vi "超标留样启动流程.vi"   [LabVIEW 2016, in "德润DR803L超标留样.lvlib"]
types:
  T1 = cluster{"采样器状态":enum16{"停止", "运行"}, "当前留样瓶编号":u16, "报警状态":enum16{"无报警", "缺水报警"}, "超标信号":enum16{"无信号", "超标信号"}, "采样器进程":enum16{"停止", "待机", "定位校正", "移除瓶盖", "采样瓶排空", "管路润洗", "管存", "进样", "瓶盖密封", "管路排空", "调整采样位置", "采样结束", "采样瓶润洗", "瓶润洗排空"}, "版本号":string, "同步信号":enum16{"无信号", "同步信号"}, "外控信号":enum16{"无信号", "外控信号"}, "门状态":enum16{"门开", "门关"}, "当前瓶号":u16, "工作状态":enum16{"停止", "采样中"}, "留样模式":enum16{"无", "定时留样", "时间等比例", "超标留样", "同步留样", "外控留样"}, "立即留样":enum16{"无", "远程留样"}, "采样方式":enum16{"单采", "双重"}, "仪器时间":timestamp, "单次采样量":u16, "时间等比采样采样间隔":u16, "排空命令":u16, "远程复位":u16, "门禁密码":u16}
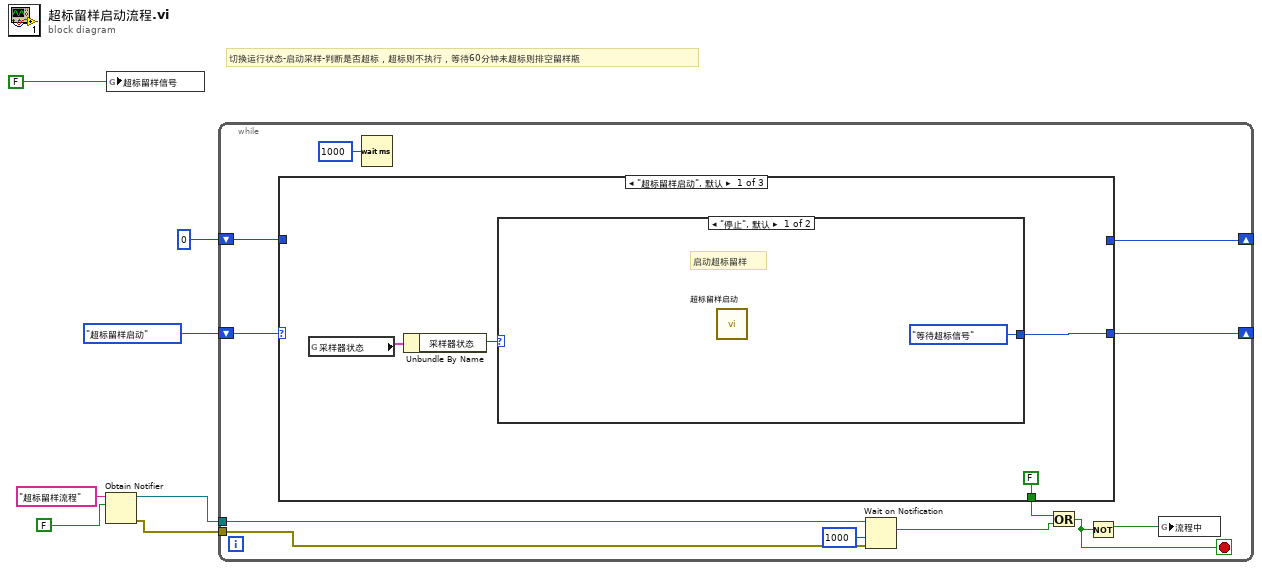
[diagram p0: block diagram]
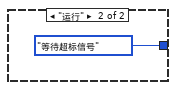
[diagram p2: hidden frame]
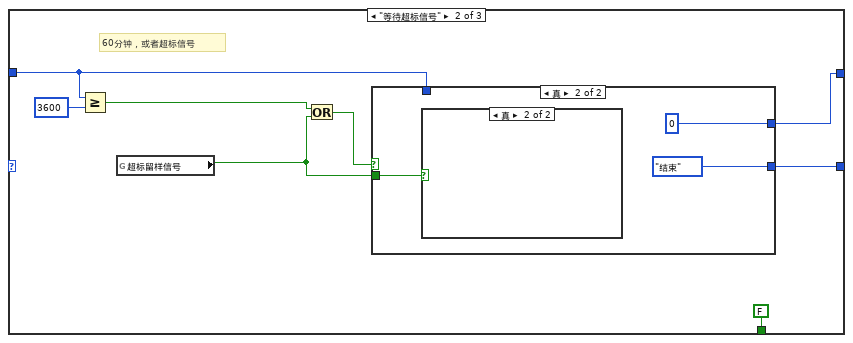
[diagram p3: hidden frame]
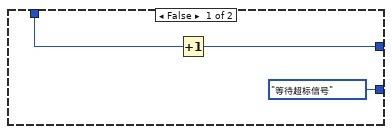
[diagram p4: hidden frame]
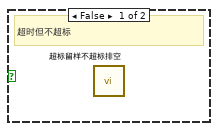
[diagram p5: hidden frame]
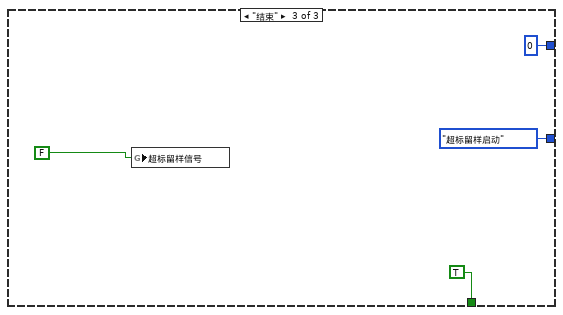
[diagram p6: hidden frame]
diagram:
  # "切换运行状态-启动采样-判断是否超标，超标则不执行，等待60分钟未超标则排空留样瓶"
  n1 = Obtain Notifier(name (unnamed)="超标留样流程" ("名称（未命名）"), notification data type=FALSE ("采样完成")) -> (notifier out=w3:refnum<notifier>, error out=w2:errorcluster)  [unwired: 2 in, 1 out]
  n2 = global write "串口参数断电保存全局变量.vi" "超标留样信号"(FALSE ("采样完成")) -> ()
  n3 = while {
    shift-right: [w10] -> _
    shift-left: enum16{"超标留样启动", "等待超标信号", "结束"}."超标留样启动" -> [w19]
    shift-right: [w16] -> _
    shift-left: 0 -> [w17]
    tunnel: w3 -> [w15]
    tunnel: w2 -> [w14]
    stop <- w12 stop-if-true
    n4 = case shown="\"超标留样启动\", 默认" w19 {
      tunnel: w17 -> [_ w29 _]
      tunnel: [_ w31 0] -> w16
      tunnel: [w21 w28 enum16{"超标留样启动", "等待超标信号", "结束"}."超标留样启动"] -> w10
      tunnel: [FALSE FALSE TRUE] -> w9
      frame "超标留样启动", Default {
        n5 = global read "超标留样全局.vi" "采样器状态"() -> (w23:T1)
        n6 = Unbundle By Name(w23) -> ("采样器状态"=w22:enum16{"停止", "运行"})
        n7 = case shown="\"停止\", 默认" w22 {
          tunnel: [enum16{"超标留样启动", "等待超标信号", "结束"}."等待超标信号" enum16{"超标留样启动", "等待超标信号", "结束"}."等待超标信号"] -> w21
          frame "停止", Default {
            # "启动超标留样"
            n8 = call "超标留样启动.vi"() -> ()  [unwired: 11 in, 1 out]
          }
          frame "运行" {
          }
        }
      }
      frame "等待超标信号" {
        # "60分钟，或者超标信号"
        n9 = Greater Or Equal?(x=w29, y=3600) -> (x >= y?=w32:bool)
        n10 = global read "串口参数断电保存全局变量.vi" "超标留样信号"() -> (w26:bool)
        n11 = Or(x=w32, y=w26) -> (x .or. y?=w30:bool)
        n12 = case shown="真" w30 {
          tunnel: [enum16{"超标留样启动", "等待超标信号", "结束"}."等待超标信号" enum16{"超标留样启动", "等待超标信号", "结束"}."结束"] -> w28
          tunnel: w29 -> [w36 _]
          tunnel: [w35 0] -> w31
          tunnel: w26 -> [_ w37]
          frame False {
            n13 = Increment(x=w36) -> (x+1=w35:i32)
          }
          frame True {
            n14 = case shown="真" w37 {
              frame False {
                # "超时但不超标"
                n15 = call "超标留样不超标排空.vi"() -> ()  [unwired: 11 in, 1 out]
              }
              frame True {
              }
            }
          }
        }
      }
      frame "结束" {
        n16 = global write "串口参数断电保存全局变量.vi" "超标留样信号"(FALSE ("采样完成")) -> ()
      }
    }
    n17 = Wait (ms)(milliseconds to wait=u32 1000 ("等待时间（毫秒）")) -> ()  [unwired: 1 out]
    n18 = Wait on Notification(notifier=w15, timeout in ms (-1)=1000 ("超时毫秒(-1)"), error in (no error)=w14) -> (notification=w11:bool)  [unwired: 1 in, 3 out]
    n19 = Or(x=w9, y=w11) -> (x .or. y?=w12:bool)
    n20 = Not(x=w12) -> (.not. x?=w8:bool)
    n21 = global write "串口参数断电保存全局变量.vi" "流程中"(w8) -> ()
  }
